vi "GenBinArrays_FASTSCAN.vi"(4 "Pixels Per Line":dbl=1024.0, 5 "FPGA Acquisition Clock Rate (MHz)":dbl=200.0, 6 "Collection Percent (%)":dbl=64.0, 7 "Scan Rate (kHz)":dbl=16.0) -> (0 "Reported Parameters":T1, 1 "Normalization Array":sgl[](array[numeric]), 2 "Pre Binned Counts (x100)":u32[](array[numeric]), 3 "FPGA Bin Edges":bool[](array[boolean]))   [LabVIEW 2016]
panel:
  out "FPGA Sampling Period (ns)":dbl
  out "Counting Period Edges (ns)":dbl[](array[numeric]) format="%#_10g"
  out "Normalized Scan Start Position":dbl
  out "Normalized Scan End Position":dbl
  out "Stop Time (us)":dbl
  out "Start Time (us)":dbl
  out "Samples Per Counting Period":i32
  out "Counting Period (us)":dbl
  # "Note that at transition points the fractional photons have been combined for data packing."
  # "Copyright (C) 2020 Edward S Allgeyer\n\nRedistribution and use in source and binary forms, with or without\nmodification, are permitted provided that the following conditions\nare met:\n\n1. Redistributions of source code must retain the above copyright\n   notice, this list of conditions and the following disclaimer.\n\n2. Redistributions in binary form must reproduce the above copyright\n   notice, this list of conditions and the following disclaimer in\n   the documentation and/or other materials provided with the\n   distribution.\n\n3. Neither the name of the copyright holder nor the names of its\n   contributors may be used to endorse or promote products derived\n   from this software without specific prior written permission.\n\nTHIS SOFTWARE IS PROVIDED BY THE COPYRIGHT HOLDERS AND CONTRIBUTORS\n\"AS IS\" AND ANY EXPRESS OR IMPLIED WARRANTIES, INCLUDING, BUT NOT\nLIMITED TO, THE IMPLIED WARRANTIES OF MERCHANTABILITY AND FITNESS\nFOR A PARTICULAR PURPOSE ARE DISCLAIMED. IN NO EVENT SHALL THE\nCOPYRIGHT HOLDER OR CONTRIBUTORS BE LIABLE FOR ANY DIRECT, INDIRECT,\nINCIDENTAL, SPECIAL, EXEMPLARY, OR CONSEQUENTIAL DAMAGES (INCLUDING,\nBUT NOT LIMITED TO, PROCUREMENT OF SUBSTITUTE GOODS OR SERVICES;\nLOSS OF USE, DATA, OR PROFITS; OR BUSINESS INTERRUPTION) HOWEVER\nCAUSED AND ON ANY THEORY OF LIABILITY, WHETHER IN CONTRACT, STRICT\nLIABILITY, OR TORT (INCLUDING NEGLIGENCE OR OTHERWISE) ARISING IN\nANY WAY OUT OF THE USE OF THIS SOFTWARE, EVEN IF ADVISED OF THE\nPOSSIBILITY OF SUCH DAMAGE."
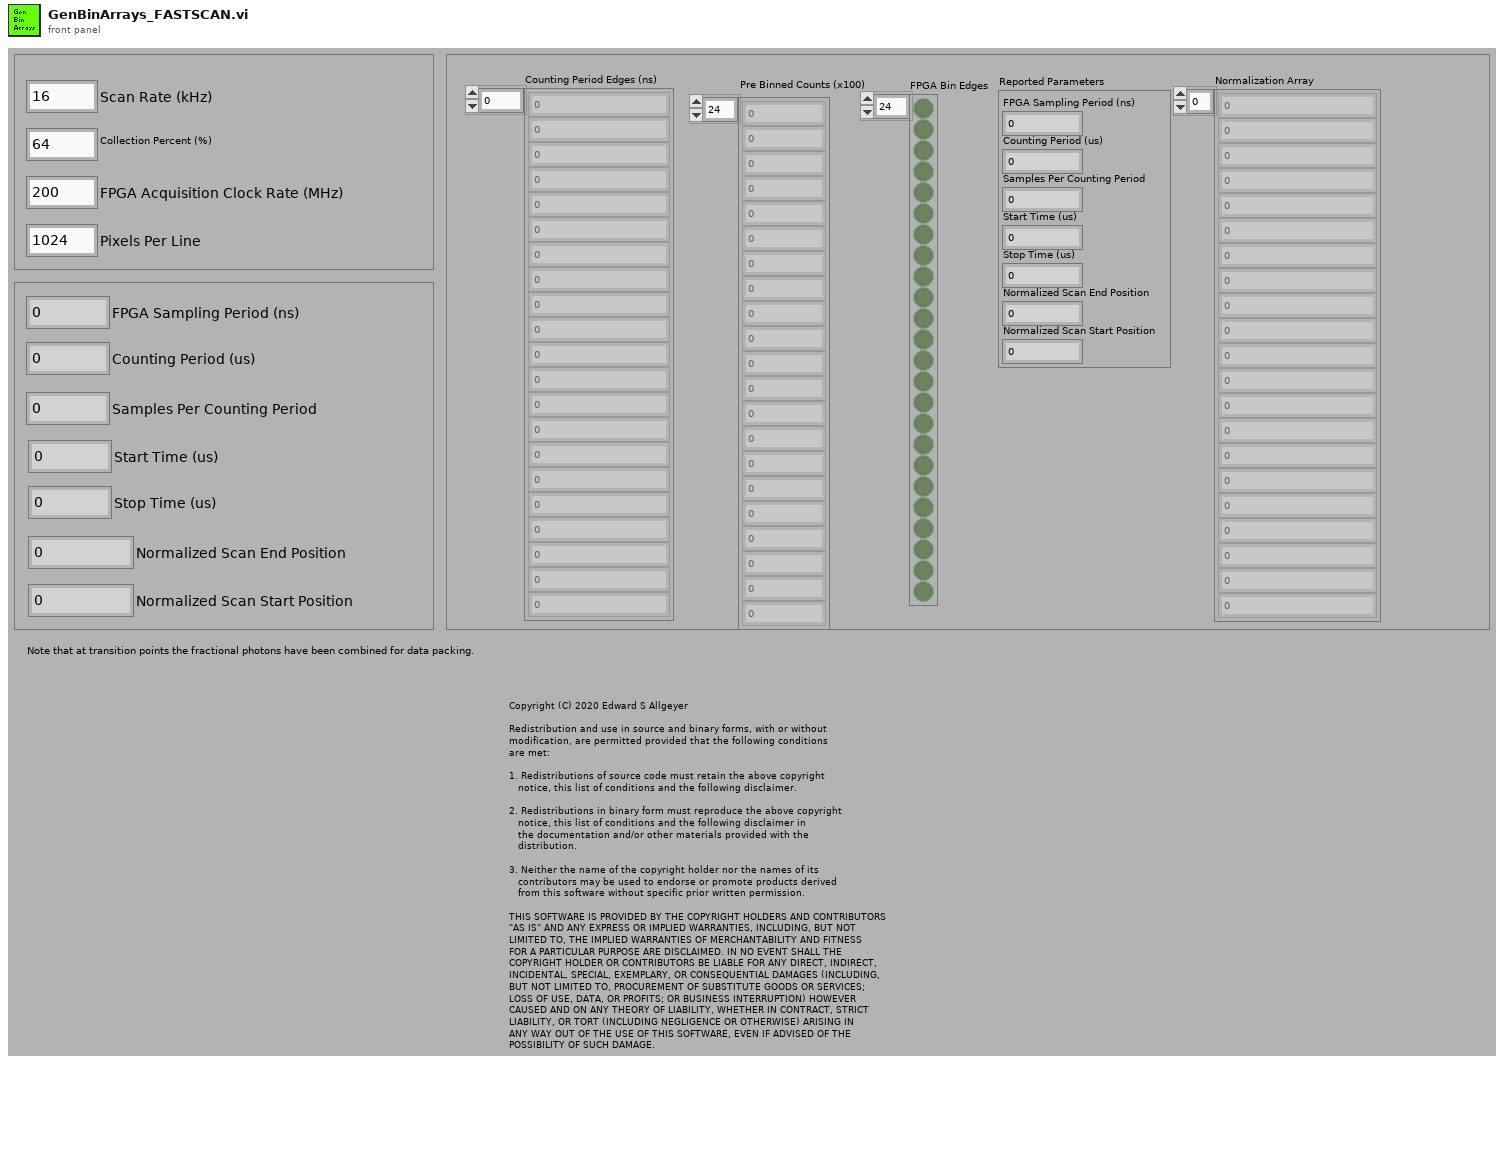
[diagram p1: front panel]
types:
  T1 = cluster{"FPGA Sampling Period (ns)":dbl, "Counting Period (us)":dbl, "Samples Per Counting Period":i32, "Start Time (us)":dbl, "Stop Time (us)":dbl, "Normalized Scan End Position":dbl, "Normalized Scan Start Position":dbl}
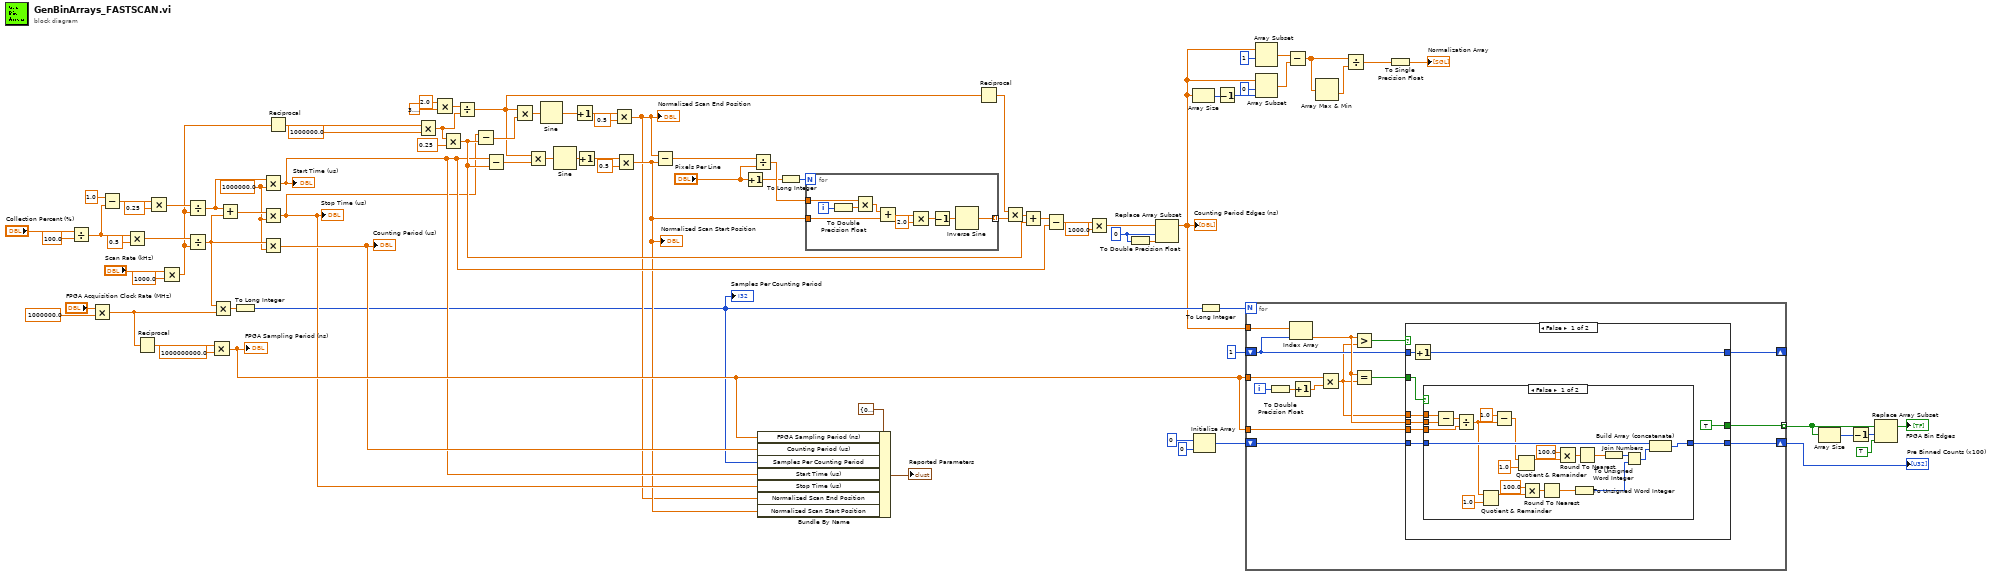
[diagram p0: block diagram]
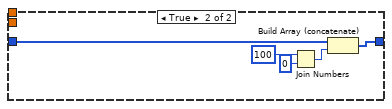
[diagram p2: hidden frame]
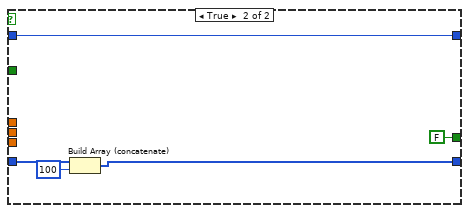
[diagram p3: hidden frame]
diagram:
  w38 = 0 ("index")
  w71 = 1000000.0 ("y")
  n1 = Divide(x="Collection Percent (%)", y=100.0) -> (x/y=w80:dbl)
  n2 = Multiply(x="FPGA Acquisition Clock Rate (MHz)", y=1000000.0) -> (x*y=w37:dbl)
  n3 = Subtract(x=1.0, y=w80) -> (x-y=w79:dbl)
  n4 = Multiply(x=w80, y=0.5) -> (x*y=w82:dbl)
  n5 = Reciprocal(x=w37) -> (1/x=w36:dbl)
  n6 = Multiply(x=w79, y=0.25) -> (x*y=w77:dbl)
  n7 = Multiply(x="Scan Rate (kHz)", y=1000.0) -> (x*y=w52:dbl)
  n8 = Divide(x=w77, y=w52) -> (x/y=w61:dbl)
  n9 = Divide(x=w82, y=w52) -> (x/y=w73:dbl)
  n10 = Multiply(x=w36, y=1000000000.0) -> (x*y=w23:dbl)
  "FPGA Sampling Period (ns)" <- w23
  n11 = Multiply(x=w73, y=w37) -> (x*y=w21:dbl)
  n12 = Add(x=w61, y=w73) -> (x+y=w72:dbl)
  n13 = To Long Integer(number=w21) -> (32bit integer=w16:i32)
  "Samples Per Counting Period" <- w16
  n14 = Multiply(x=w61, y=w71) -> (x*y=w20:dbl)
  "Start Time (us)" <- w20
  n15 = Multiply(x=w72, y=w71) -> (x*y=w19:dbl)
  "Stop Time (us)" <- w19
  n16 = Multiply(x=w73, y=w71) -> (x*y=w22:dbl)
  "Counting Period (us)" <- w22
  n17 = Reciprocal(x=w52) -> (1/x=w59:dbl)
  n18 = Multiply(x=w59, y=1000000.0) -> (x*y=w58:dbl)
  n19 = Multiply(x=2.0 ("y"), y=3.141592653589793) -> (x*y=w67:dbl)
  n20 = Multiply(x=w58, y=0.25) -> (x*y=w44:dbl)
  n21 = Divide(x=w67, y=w58) -> (x/y=w48:dbl)
  n22 = Subtract(x=w19, y=w44) -> (x-y=w66:dbl)
  n23 = Subtract(x=w20, y=w44) -> (x-y=w53:dbl)
  n24 = Multiply(x=w48, y=w66) -> (x*y=w65:dbl)
  n25 = Multiply(x=w48, y=w53) -> (x*y=w54:dbl)
  n26 = Sine(x=w65) -> (sin(x)=w64:dbl)
  n27 = Sine(x=w54) -> (sin(x)=w55:dbl)
  n28 = Increment(x=w64) -> (x+1=w63:dbl)
  n29 = Increment(x=w55) -> (x+1=w56:dbl)
  n30 = Multiply(x=w63, y=0.5) -> (x*y=w17:dbl)
  "Normalized Scan End Position" <- w17
  n31 = Multiply(x=w56, y=0.5) -> (x*y=w18:dbl)
  "Normalized Scan Start Position" <- w18
  n32 = Subtract(x=w17, y=w18) -> (x-y=w51:dbl)
  n33 = Increment(x="Pixels Per Line") -> (x+1=w25:dbl)
  n34 = Divide(x=w51, y="Pixels Per Line") -> (x/y=w50:dbl)
  n35 = Bundle By Name(cluster=T1 {"FPGA Sampling Period (ns)"=0.0, "Counting Period (us)"=0.0, "Samples Per Counting Period"=0, "Start Time (us)"=0.0, "Stop Time (us)"=0.0, "Normalized Scan End Position"=0.0, "Normalized Scan Start Position"=0.0}, "FPGA Sampling Period (ns)"=w23, "Counting Period (us)"=w22, "Samples Per Counting Period"=w16, "Start Time (us)"=w20, "Stop Time (us)"=w19, "Normalized Scan End Position"=w17, "Normalized Scan Start Position"=w18) -> (→"Reported Parameters":T1)
  n36 = To Long Integer(number=w25) -> (32bit integer=w49:i32)
  n37 = for {
    N: w49 -> [_]
    tunnel: w18 -> [w96]
    tunnel: w50 -> [w95]
    tunnel: [w88] -> w47 mode=indexing
    i -> [w94]
    n38 = To Double Precision Float(number=w94) -> (double precision float=w93:dbl)
    n39 = Multiply(x=w95, y=w93) -> (x*y=w92:dbl)
    n40 = Add(x=w92, y=w96) -> (x+y=w87:dbl)
    n41 = Multiply(x=w87, y=2.0) -> (x*y=w90:dbl)
    n42 = Decrement(x=w90) -> (x-1=w89:dbl)
    n43 = Inverse Sine(1:w89) -> (0:w88:dbl)
  }
  n44 = Reciprocal(x=w48) -> (1/x=w46:dbl)
  n45 = Multiply(x=w46, y=w47) -> (x*y=w45:dbl[])
  n46 = Add(x=w45, y=w44) -> (x+y=w43:dbl[])
  n47 = Subtract(x=w43, y=w20) -> (x-y=w42:dbl[])
  n48 = Multiply(x=w42, y=1000.0) -> (x*y=w40:dbl[])
  n49 = To Double Precision Float(number=w38) -> (double precision float=w39:dbl)
  n50 = Replace Array Subset(array=w40, new element=w39, index=w38) -> (w8:dbl[])
  "Counting Period Edges (ns)" <- w8
  n51 = Array Size(array=w8) -> (size(s)=w14:i32)
  n52 = Initialize Array(u32 0 ("element"), 0 ("dimension size")) -> (w31:u32[])
  n53 = To Long Integer(number=w16) -> (32bit integer=w15:i32)
  n54 = Decrement(x=w14) -> (x-1=w12:i32)
  n55 = for {
    N: w15 -> [_]
    tunnel: w23 -> [w108]
    tunnel: w8 -> [w111]
    shift-right: [w99] -> _
    shift-left: 1 ("index") -> [w100]
    shift-right: [w104] -> w2
    shift-left: w31 -> [w105]
    tunnel: w23 -> [w102]
    tunnel: [w98] -> w27 mode=indexing
    i -> [w109]
    n56 = To Double Precision Float(number=w109) -> (double precision float=w110:dbl)
    n57 = Index Array(array=w111, index=w100) -> (element=w103:dbl)
    n58 = Increment(x=w110) -> (x+1=w107:dbl)
    n59 = Multiply(x=w108, y=w107) -> (x*y=w97:dbl)
    n60 = Greater?(x=w103, y=w97) -> (0:w106:bool)
    n61 = Equal?(x=w103, y=w97) -> (x = y?=w101:bool)
    n62 = case shown="False" w106 {
      tunnel: w105 -> [w117 w152]
      tunnel: [w116 w150] -> w104
      tunnel: [TRUE FALSE] -> w98
      tunnel: w97 -> [w120 _]
      tunnel: w103 -> [w119 _]
      tunnel: w102 -> [w118 _]
      tunnel: w101 -> [w112 _]
      tunnel: w100 -> [w114 w148]
      tunnel: [w113 w148] -> w99
      frame False {
        n63 = Increment(x=w114) -> (x+1=w113:i32)
        n64 = case shown="False" w112 {
          tunnel: w120 -> [w141 _]
          tunnel: w119 -> [w140 _]
          tunnel: w118 -> [w139 _]
          tunnel: w117 -> [w137 w147]
          tunnel: [w136 w146] -> w116
          frame False {
            n65 = Subtract(x=w141, y=w140) -> (x-y=w142:dbl)
            n66 = Divide(x=w142, y=w139) -> (x/y=w131:dbl)
            n67 = Quotient & Remainder(x=w131, y=1.0) -> (x-y*floor(x/y)=w133:dbl)  [unwired: 1 out]
            n68 = Subtract(x=1.0, y=w131) -> (x-y=w124:dbl)
            n69 = Quotient & Remainder(x=w124, y=1.0) -> (x-y*floor(x/y)=w127:dbl)  [unwired: 1 out]
            n70 = Multiply(x=100.0, y=w133) -> (x*y=w135:dbl)
            n71 = Round To Nearest(number=w135) -> (nearest integer value=w130:dbl)
            n72 = Multiply(x=100.0, y=w127) -> (x*y=w125:dbl)
            n73 = To Unsigned Word Integer(number=w130) -> (unsigned 16bit integer=w122:u16)
            n74 = Round To Nearest(number=w125) -> (nearest integer value=w129:dbl)
            n75 = To Unsigned Word Integer(number=w129) -> (unsigned 16bit integer=w123:u16)
            n76 = Join Numbers(hi=w123, lo=w122) -> ((hi.lo)=w121:u32)
            n77 = Build Array (concatenate)(w137, w121) -> (w136:u32[])
          }
          frame True {
            n78 = Join Numbers(hi=u16 100, lo=u16 0) -> ((hi.lo)=w143:u32)
            n79 = Build Array (concatenate)(w147, w143) -> (w146:u32[])
          }
        }
      }
      frame True {
        n80 = Build Array (concatenate)(w152, u32 100) -> (w150:u32[])
      }
    }
  }
  "Pre Binned Counts (x100)" <- w2
  n81 = Array Subset(array=w8, index=1) -> (w10:dbl[])  [unwired: 1 in]
  n82 = Array Subset(array=w8, index=0, length=w12) -> (w9:dbl[])
  n83 = Subtract(x=w10, y=w9) -> (x-y=w7:dbl[])
  n84 = Array Max & Min(array=w7) -> (min value=w6:dbl)  [unwired: 3 out]
  n85 = Divide(x=w7, y=w6) -> (x/y=w5:dbl[])
  n86 = To Single Precision Float(number=w5) -> (single precision float=→"Normalization Array":sgl[])
  n87 = Array Size(array=w27) -> (size(s)=w30:i32)
  n88 = Decrement(x=w30) -> (x-1=w29:i32)
  n89 = Replace Array Subset(array=w27, new element=TRUE, index=w29) -> (→"FPGA Bin Edges":bool[])
